vi "Write.vi"(8 "error in (no error)":errorcluster, 10 "Value":T1, 11 "Double Float.lvclass in":refnum<class "Abs_U8 Integer 1D.lvclass">) -> (0 "error out":errorcluster, 3 "Double Float.lvclass out":refnum<class "Abs_U8 Integer 1D.lvclass">)   [LabVIEW 2021, in "Abs_U8 Integer 1D.lvclass"]
uses:
  Abs_U8 Integer 1D.lvclass
  Support/Type.ctl
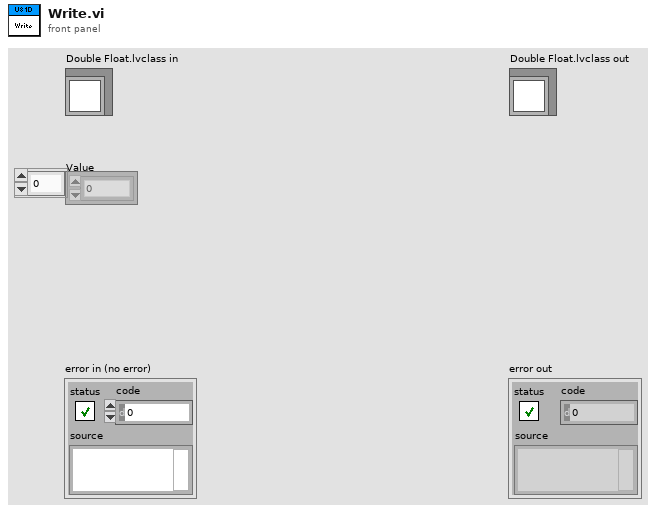
[diagram p1: front panel]
types:
  T1 = typedef "Abs_U8 Integer 1D.lvclass/Type.ctl" = u8[]
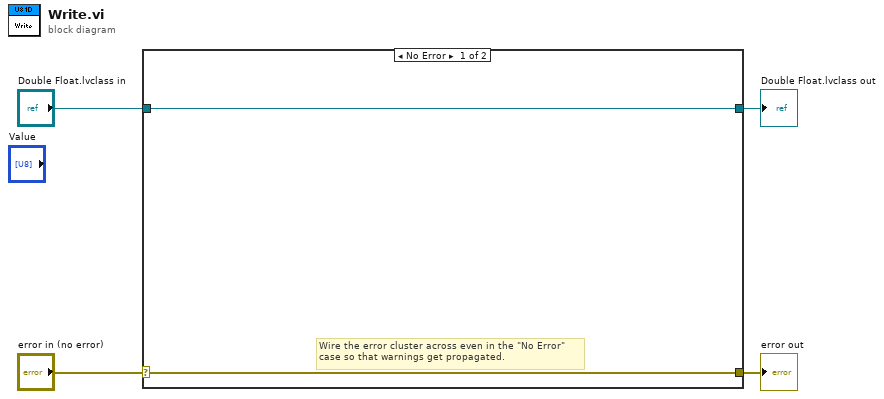
[diagram p0: block diagram]
diagram:
  n1 = case shown="No Error" "error in (no error)" {
    selector: "error in (no error)" -> [w5 w8]
    tunnel: [w5 w8] -> w3
    tunnel: [w6 w7] -> w1
    tunnel: "Double Float.lvclass in" -> [w6 w7]
    frame No Error {
      # "Wire the error cluster across even in the \"No Error\"\ncase so that warnings get propagated."
    }
    frame Error {
    }
  }
  "error out" <- w3
  "Double Float.lvclass out" <- w1
